vi "Find Latest Folder of Images.vi"(8 "Error In":errorcluster) -> (0 "error out":errorcluster, 3 "Latest Folder of Images":string)   [LabVIEW 2014]
uses:
  Controls/Folders of Images on RedEdge.ctl
  <vilib>/httpClient/LabVIEWHTTPClient.lvlib
panel:
  out "directories 2":string[](array[string])
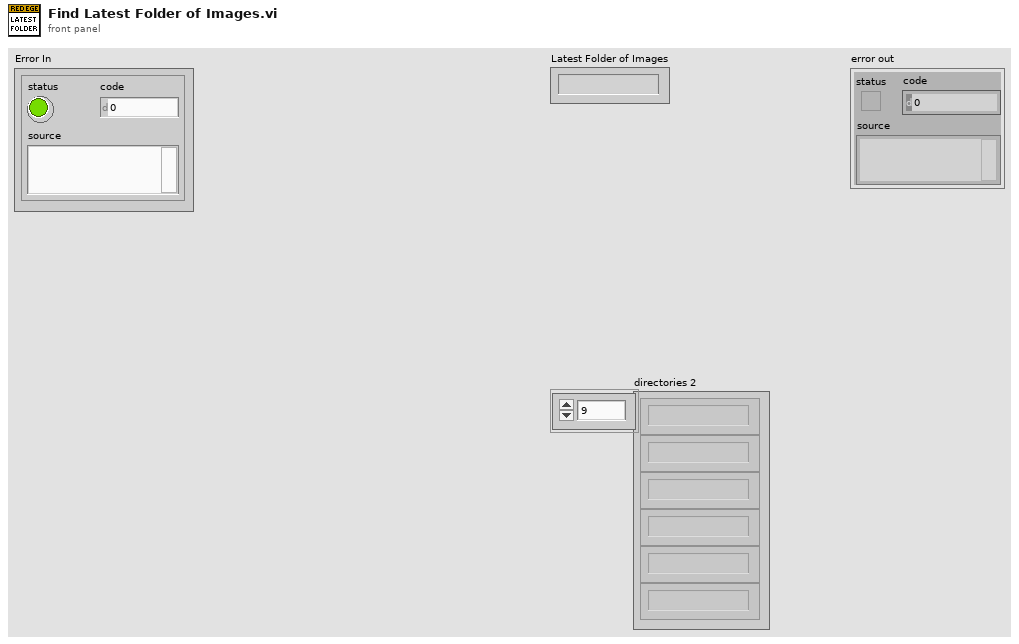
[diagram p1: front panel]
types:
  T1 = typedef "Folders of Images on RedEdge.ctl" = cluster{"directories":string[]}
  T2 = typedef "LabVIEWHTTPClient.lvlib/ClientHandle.ctl" = refnum<k1>
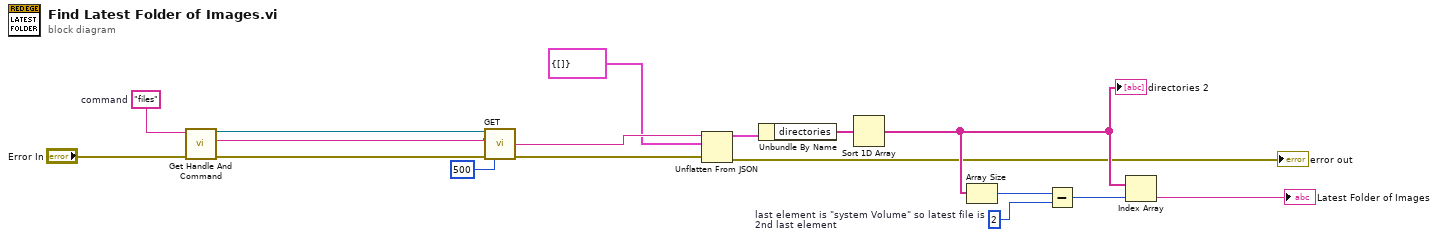
[diagram p0: block diagram]
diagram:
  w4 = 2  # last element is "system Volume" so latest file is 2nd last element
  w17 = "files"  # command
  n1 = call "Get Handle And Command.vi"("Error In"="Error In", "Command"=w17) -> ("Error Out"=w15:errorcluster, "Command URL"=w14:string, "RedEdge client handle out"=w16:T2)  [unwired: 6 in]
  n2 = call <vilib>:"GET.vi"("client handle"=w16, "url"=w14, "error in (no error)"=w15, "timeout (10000)"=500) -> ("body"=w13:string, "error out"=w9:errorcluster)  [unwired: 8 in, 2 out]
  n3 = Unflatten From JSON(JSON string=w13, type and defaults=T1 {"directories"=[]} ("Folders of Images on RedEdge"), error in (no error)=w9) -> (value=w11:T1, error out=→"error out":errorcluster)  [unwired: 4 in]
  n4 = Unbundle By Name(w11) -> ("directories"=w8:string[])
  n5 = Sort 1D Array(array=w8) -> (sorted array=w7:string[])
  "directories 2" <- w7
  n6 = Array Size(array=w7) -> (size(s)=w5:i32)
  n7 = Subtract(x=w5, y=w4) -> (x-y=w3:i32)
  n8 = Index Array(array=w7, index=w3) -> (element=→"Latest Folder of Images":string)
